vi "Initialize.vi"(8 "error in (no error)":errorcluster, 11 "device data model in":refnum<class "ICPCON ET Data Model.lvclass">) -> (0 "error out":errorcluster, 3 "device data model out":refnum<class "ICPCON ET Data Model.lvclass">)   [LabVIEW 2021, in "ICPCON ET Data Model.lvclass"]
doc: "This VI initializes the device data model."
uses:
  ICPCON ET Data Model.lvclass
  Type Definitions/Data Model.ctl
  ICPCON ET Data Model.lvclass/ICPCON ET Data Model.ctl
  Modbus_v121c/Data Model/Device Data Model.lvclass
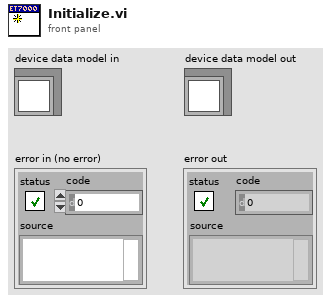
[diagram p1: front panel]
types:
  T1 = typedef "ICPCON ET Data Model.lvclass/Data Model.ctl" = cluster{"UTC":u64, "DI":bool[], "DO":bool[], "IR":u16[], "HR":u16[], "ES":u8}
  T2 = typedef "Device Data Model.lvclass/N channel.ctl" = cluster{"N DI channel":i32, "N DO channel":i32, "N AI channel":i32, "N AO channel":i32}
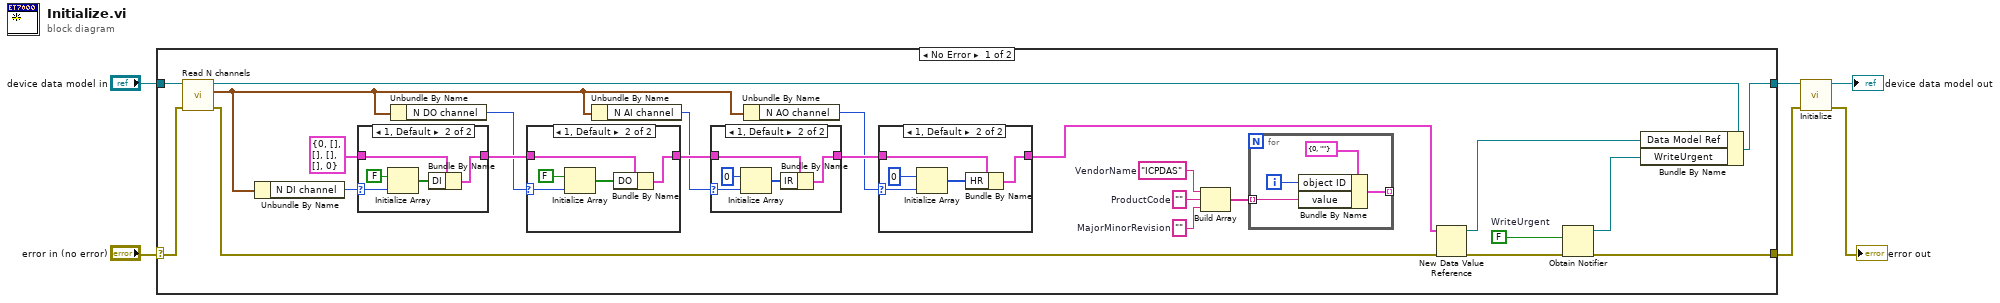
[diagram p0: block diagram]
diagram:
  n1 = case shown="No Error" "error in (no error)" {
    selector: "error in (no error)" -> [w18 w59]
    tunnel: "device data model in" -> [w19 w60]
    tunnel: [w7 w59] -> w5
    tunnel: [w26 w60] -> w4
    frame No Error {
      w10 = FALSE  # WriteUrgent
      w28 = ""  # MajorMinorRevision
      w30 = ""  # ProductCode
      w29 = "ICPDAS"  # VendorName
      n2 = call-dynamic "Read N channels.vi"("error in (no error)"=w18, "device data model in"=w19) -> ("error out"=w17:errorcluster, "N channel"=w12:T2, "device data model out"=w20:refnum<class "ICPCON ET Data Model.lvclass">)  [unwired: 7 in]
      n3 = Unbundle By Name(w12) -> ("N DI channel"=w15:i32)
      n4 = case shown="1, Default" w15 {
        selector: w15 -> [_ w38]
        tunnel: T1 {"UTC"=0, "DI"=[], "DO"=[], "IR"=[], "HR"=[], "ES"=0} ("Data Model") -> [w37 w41]
        tunnel: [w37 w39] -> w24
        frame 0 {
        }
        frame 1, Default {
          n5 = Initialize Array(FALSE ("Boolean"), w38) -> (w40:bool[])
          n6 = Bundle By Name(cluster=w41, "DI"=w40) -> (w39:T1)
        }
      }
      n7 = Unbundle By Name(w12) -> ("N DO channel"=w14:i32)
      n8 = case shown="1, Default" w14 {
        selector: w14 -> [_ w33]
        tunnel: w24 -> [w31 w36]
        tunnel: [w31 w34] -> w22
        frame 0 {
        }
        frame 1, Default {
          n9 = Initialize Array(FALSE ("Boolean"), w33) -> (w35:bool[])
          n10 = Bundle By Name(cluster=w36, "DO"=w35) -> (w34:T1)
        }
      }
      n11 = Unbundle By Name(w12) -> ("N AI channel"=w13:i32)
      n12 = case shown="1, Default" w13 {
        selector: w13 -> [_ w51]
        tunnel: w22 -> [w49 w54]
        tunnel: [w49 w52] -> w23
        frame 0 {
        }
        frame 1, Default {
          n13 = Initialize Array(u16 0, w51) -> (w53:u16[])
          n14 = Bundle By Name(cluster=w54, "IR"=w53) -> (w52:T1)
        }
      }
      n15 = Unbundle By Name(w12) -> ("N AO channel"=w11:i32)
      n16 = case shown="1, Default" w11 {
        selector: w11 -> [_ w45]
        tunnel: w23 -> [w43 w48]
        tunnel: [w43 w46] -> w21
        frame 0 {
        }
        frame 1, Default {
          n17 = Initialize Array(u16 0, w45) -> (w47:u16[])
          n18 = Bundle By Name(cluster=w48, "HR"=w47) -> (w46:T1)
        }
      }
      n19 = Build Array(w29, w30, w28) -> (w27:string[])
      n20 = for {
        tunnel: w27 -> [w56] mode=indexing
        tunnel: [w55] -> _ mode=indexing
        i -> [w57]
        n21 = Bundle By Name(cluster=cluster{"object ID":u8, "value":string} {"object ID"=0, "value"=""} ("Cluster"), "object ID"=w57, "value"=w56) -> (w55:cluster{"object ID":u8, "value":string})
      }
      n22 = New Data Value Reference(data value=w21, error in=w17) -> (data value reference=w25:refnum<data-value>, error out=w9:errorcluster)
      n23 = Obtain Notifier(notification data type=w10, error in (no error)=w9) -> (notifier out=w8:refnum<notifier>, error out=w7:errorcluster)  [unwired: 2 in, 1 out]
      n24 = Bundle By Name(cluster=w20, "Data Model Ref"=w25, "WriteUrgent"=w8) -> (w26:refnum<class "ICPCON ET Data Model.lvclass">)
    }
    frame Error {
    }
  }
  n25 = call-parent "Initialize.vi"("error in"=w5, "device data model in"=w4) -> ("error out"=→"error out":errorcluster, "device data model out"=→"device data model out":refnum<class "ICPCON ET Data Model.lvclass">)  [unwired: 8 in]
